vi "server address.vi"() -> (3 "Server Address":string)   [LabVIEW 2024]
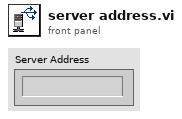
[diagram p1: front panel]
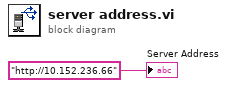
[diagram p0: block diagram]
diagram:
  "Server Address" <- "http://10.152.236.66" ("Server Address")
